vi "tsapp_set_flexray_channel_count.vi"(8 "error in (no error)":errorcluster caption="错误输入（无错误）", 10 "ACount":i32, 11 "path in":path) -> (0 "error out":errorcluster caption="错误输出", 2 "function return":i32, 3 "path out":path)   [LabVIEW 2014]
doc: "TSAPI(s32)tsapp_set_flexray_channel_count(const s32 ACount);"
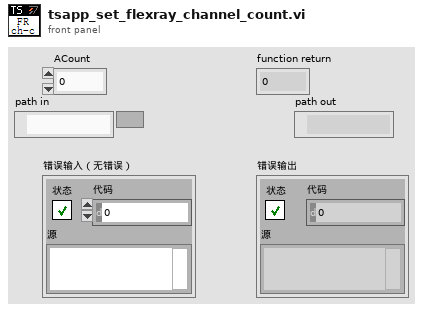
[diagram p1: front panel]
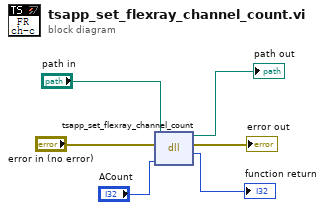
[diagram p0: block diagram]
diagram:
  n1 = dll-call lib="D:/Work/LabVIEW Code/TSMaster Labview SDK/LabVIEW/LabVIEW-TSMasterAPI_CLN/TSMasterAPI_LabVIEW-2024-10-08 14-20-13/Not_organized_vi/TSMaster.*" fn="tsapp_set_flexray_channel_count"(path in="path in", error in="error in (no error)", "ACount"="ACount") -> (path out=→"path out":path, error out=→"error out":errorcluster, "返回类型"=→"function return":i32)  [unwired: 2 in]
